vi "Find Controllers.vi"(8 "error in (no error)":errorcluster) -> (0 "error out":errorcluster, 2 "Controllers":string[](array[string]), 3 "COM ports":string[](array[string]))   [LabVIEW 2017]
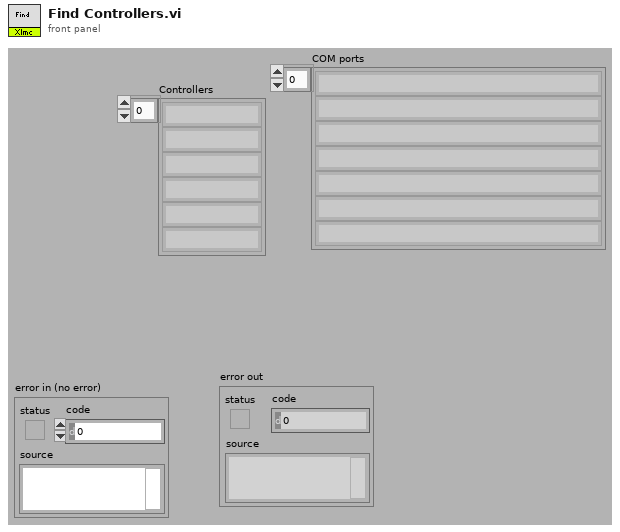
[diagram p1: front panel]
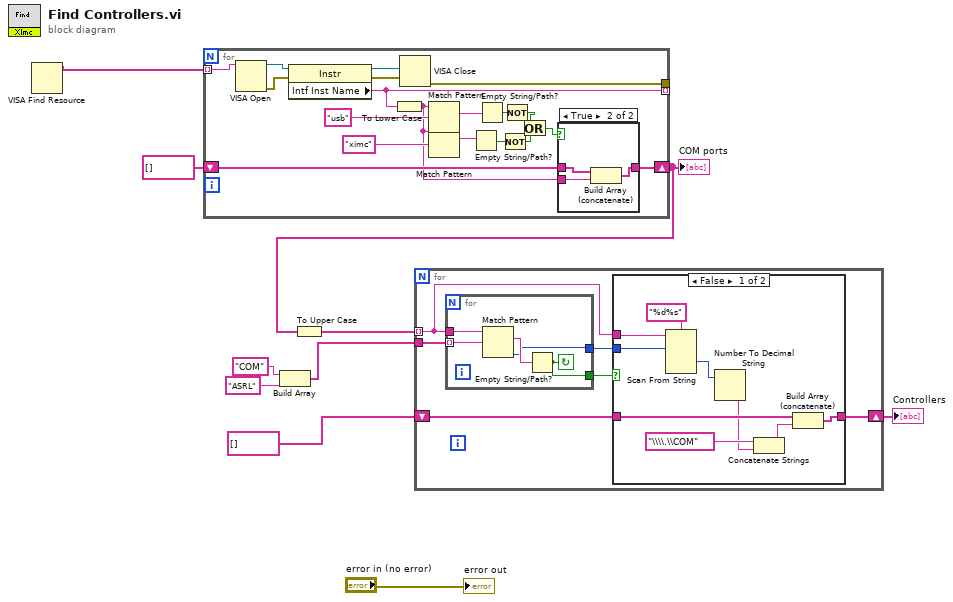
[diagram p0: block diagram]
diagram:
  n1 = VISA Find Resource() -> (3:w5:string[])  [unwired: 3 in, 2 out]
  n2 = for {
    tunnel: w5 -> [w19] mode=indexing
    tunnel: [w25] -> _ mode=indexing
    shift-right: [w21] -> w3
    shift-left: string[] [] -> [w22]
    tunnel: [w18] -> _
    n3 = VISA Open(VISA resource name=w19) -> (VISA resource name=w29:refnum<visa-resource-name>, error out=w28:errorcluster)  [unwired: 4 in]
    n4 = property class="Instr"(reference=w29, error in=w28) -> (reference out=w27:refnum<visa-resource-name>, error out=w26:errorcluster, "Intf Inst Name"=w25:string)
    n5 = To Lower Case(string=w25) -> (all lower case string=w11:string)
    n6 = VISA Close(VISA resource name=w27, error in (no error)=w26) -> (error out=w18:errorcluster)
    n7 = Match Pattern(string=w11, regular expression="usb") -> (match substring=w20:string)  [unwired: 1 in, 3 out]
    n8 = Match Pattern(string=w11, regular expression="ximc") -> (match substring=w16:string)  [unwired: 1 in, 3 out]
    n9 = Empty String/Path?(string/path=w16) -> (empty?=w15:bool)
    n10 = Empty String/Path?(string/path=w20) -> (empty?=w23:bool)
    n11 = Not(x=w15) -> (.not. x?=w12:bool)
    n12 = Not(x=w23) -> (.not. x?=w13:bool)
    n13 = Or(x=w13, y=w12) -> (x .or. y?=w14:bool)
    n14 = case shown="True" w14 {
      tunnel: w22 -> [w30 w33]
      tunnel: [w30 w32] -> w21
      tunnel: w11 -> [_ w31]
      frame False {
      }
      frame True {
        n15 = Build Array (concatenate)(w33, w31) -> (w32:string[])
      }
    }
  }
  "COM ports" <- w3
  n16 = Build Array("COM" ("regular expression"), "ASRL" ("regular expression")) -> (w7:string[])
  n17 = To Upper Case(1:w3) -> (0:w10:string[])
  n18 = for {
    tunnel: w10 -> [w36] mode=indexing
    tunnel: w7 -> [w39]
    shift-right: [w34] -> w2
    shift-left: string[] [] -> [w35]
    n19 = for {
      tunnel: w36 -> [w54]
      tunnel: w39 -> [w53] mode=indexing
      tunnel: [w51] -> w37
      tunnel: [w50] -> w38
      stop <- w50 continue-if-true
      n20 = Match Pattern(string=w54, regular expression=w53) -> (match substring=w52:string, offset past match=w51:i32)  [unwired: 1 in, 2 out]
      n21 = Empty String/Path?(string/path=w52) -> (empty?=w50:bool)
    }
    n22 = case shown="False" w38 {
      tunnel: w37 -> [w47 _]
      tunnel: w36 -> [w48 _]
      tunnel: w35 -> [w45 w49]
      tunnel: [w44 w49] -> w34
      frame False {
        n23 = Scan From String(format string="%d%s", input string=w48, initial scan location=w47) -> (output 1=w43:i32)  [unwired: 4 in, 3 out]
        n24 = Number To Decimal String(number=w43) -> (decimal integer string=w41:string)  [unwired: 1 in]
        n25 = Concatenate Strings("\\\\.\\COM" ("name"), w41) -> (w40:string)
        n26 = Build Array (concatenate)(w45, w40) -> (w44:string[])
      }
      frame True {
      }
    }
  }
  "Controllers" <- w2
  "error out" <- "error in (no error)"
